vi "Open Deployable Source Distribution.vi"(8 "error in (no error)":errorcluster, 10 "Build specification name":string, 11 "TargetItem Refnum":refnum<vi>) -> (0 "error out":errorcluster, 3 "DSDIST out":refnum<class "NI_AB_API_DSDIST.lvclass">)   [LabVIEW 2020, in "NI_AB_API_DSDIST.lvclass"]
uses:
  <vilib>/AppBuilder/AB_API/DSDIST/NI_AB_API_DSDIST.lvclass
  e:/builds/penguin/labview/branches/2020/dev/dist/vi.lib/AppBuilder/AB_API/Build/NI_AB_API_Build.lvclass
  <vilib>/AppBuilder/AB_API/common/AB_API Build Object Type.ctl
  <vilib>/AppBuilder/AB_Classes/Build/AB_Build.lvclass
  <vilib>/AppBuilder/AB_API/Build/NI_AB_API_Build.lvclass
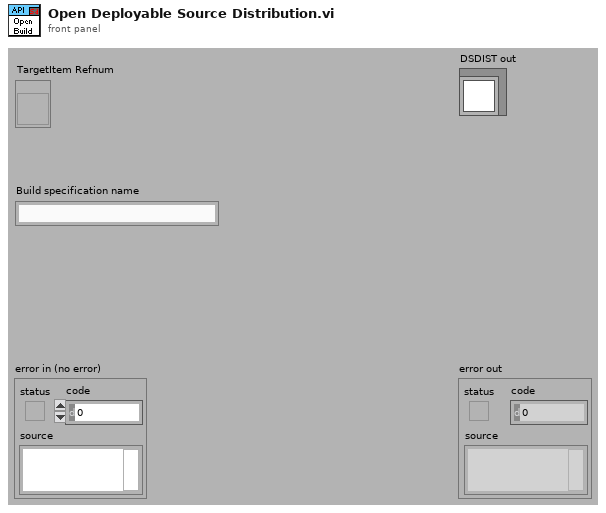
[diagram p1: front panel]
types:
  T1 = typedef "AB_API Build Object Type.ctl" = enum16{"Source Distribution", "DLL", "EXE", "Installer", "Zip File", "RESTful WS", "RTEXE", "Packed Library", "C Generation ", ".NET Interop Assembly"}
  T2 = typedef "ItemRef.ctl" = u64
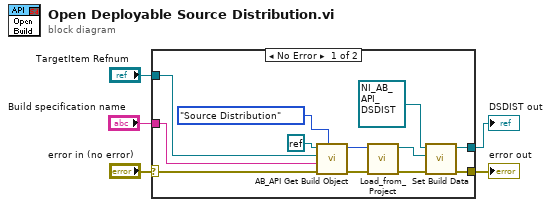
[diagram p0: block diagram]
diagram:
  n1 = case shown="No Error" "error in (no error)" {
    selector: "error in (no error)" -> [w14 w18]
    tunnel: [w9 w18] -> w4
    tunnel: [w8 _] -> w3
    tunnel: "TargetItem Refnum" -> [w17 _]
    tunnel: "Build specification name" -> [w16 _]
    frame No Error {
      n2 = call <vilib>:"AB_API Get Build Object.vi"("Build object type"=AB_API_Build_Object_Type."Source Distribution", "error in (no error)"=w14, "Build spec name"=w16, "TargetItem Refnum"=w17, "Project Refnum"=refnum<k0> refnum) -> ("error out"=w12:errorcluster, "Build Object"=w13:T2)  [unwired: 5 in]
      n3 = call <vilib>:"Load_from_Project.vi"("error in (no error)"=w12, "Object"=w13) -> ("error out"=w10:errorcluster, "Build out"=w6:refnum<class "AB_Build.lvclass">)  [unwired: 8 in]
      n4 = call <vilib>:"Set Build Data.vi"("error in (no error)"=w10, "AB_Build.lvclass"=w6, "NI_AB_API_Build in"=refnum<class "NI_AB_API_DSDIST.lvclass"> refnum ("NI_AB_API_SDIST.lvclass")) -> ("error out"=w9:errorcluster, "NI_AB_API_Build out"=w8:refnum<class "NI_AB_API_DSDIST.lvclass">)  [unwired: 7 in]
    }
    frame Error {
    }
  }
  "error out" <- w4
  "DSDIST out" <- w3
